vi "SC_schleife_init.vi"   [LabVIEW 2016]
uses:
  Oxford Software/Oxsoft/RAMP.LLB/RampTState.ctl
  Global/Global Variables/global.vi
  Global/Global Variables/Data_Display_global.vi
  Instrument_Setup.vi
types:
  T1 = typedef "RampTState.ctl" = enum16{"START", "RUN"}
  T2 = cluster{"ControlTITC":i8, "ControlTCh":i8, "SampleTITC":i8, "SampleTCh":i8}
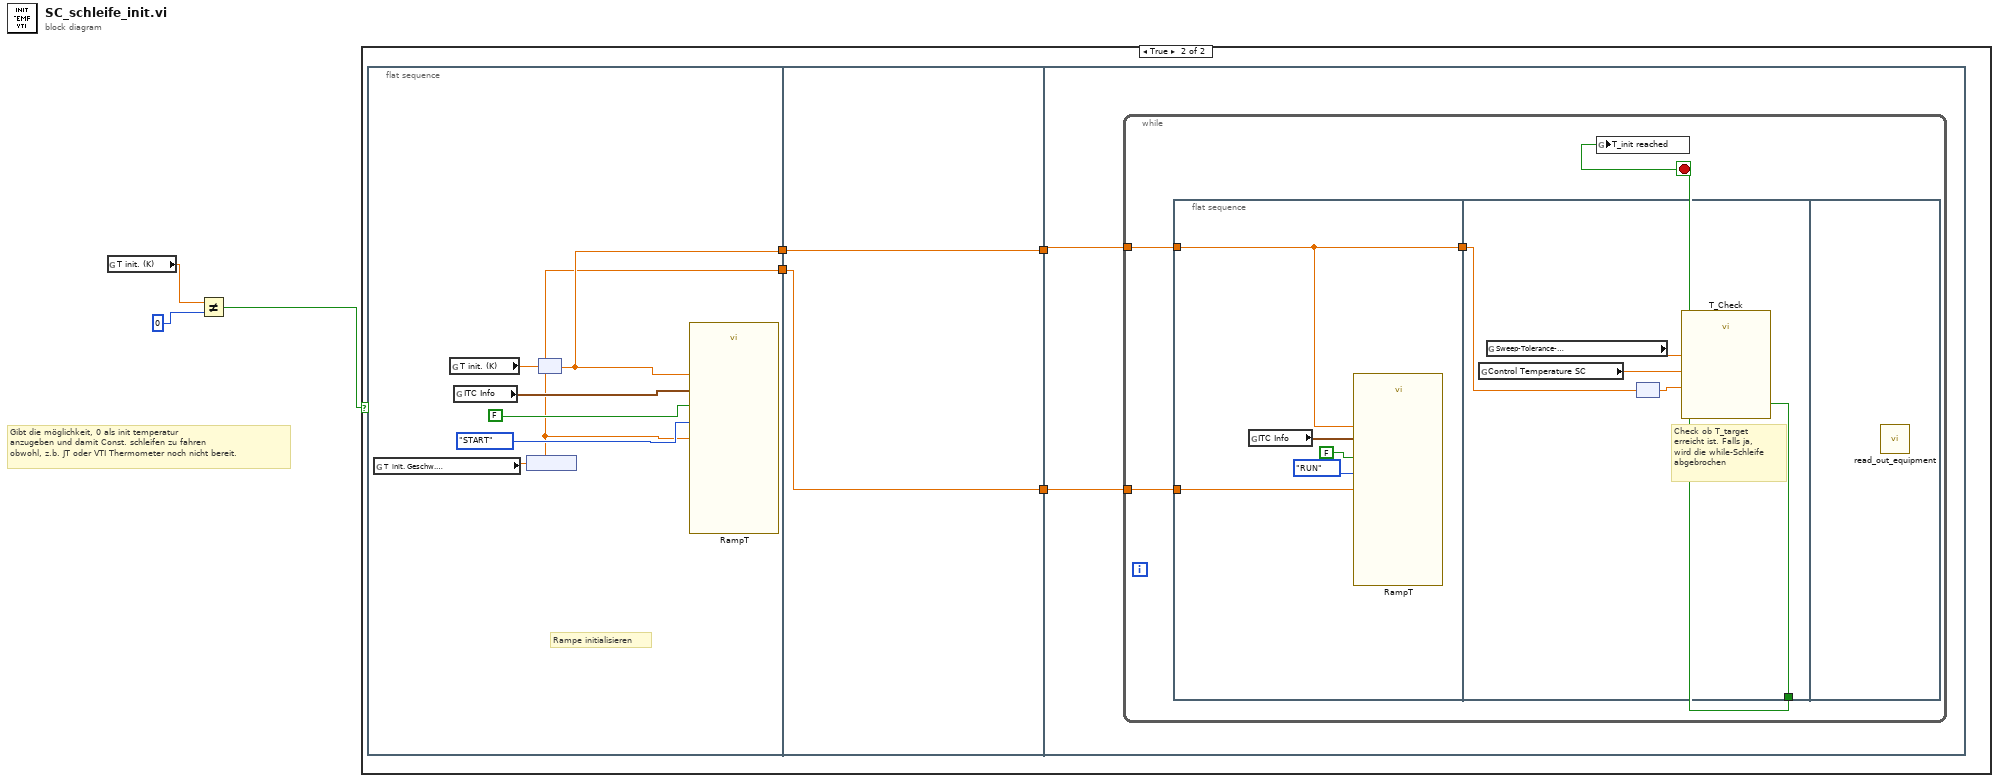
[diagram p0: block diagram]
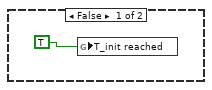
[diagram p2: hidden frame]
diagram:
  # "Gibt die möglichkeit, 0 als init temperatur \nanzugeben und damit Const. schleifen zu fahren\nobwohl, z.b. JT oder VTI Thermometer noch nicht bereit."
  n1 = global read "global.vi" "T init. (K)"() -> (w3:dbl)
  n2 = Not Equal?(x=w3, y=0) -> (x != y?=w1:bool)
  n3 = case shown="True" w1 {
    frame False {
      n4 = global write "Data_Display_global.vi" "T_init reached"(TRUE) -> ()
    }
    frame True {
      n5 = flat-sequence {
        tunnel: [w9] -> w8
        tunnel: [w10] -> w7
        tunnel: w8 -> [w16]
        tunnel: w7 -> [w17]
        tunnel: [w17] -> w6
        tunnel: [w16] -> w5
        tunnel: w6 -> [w19]
        tunnel: w5 -> [w18]
        frame #0 {
          # "Rampe initialisieren"
          n6 = global read "global.vi" "T  init. Geschw. \n(K/min)"() -> (w15:dbl)
          n7 = global read "global.vi" "T init. (K)"() -> (w14:dbl)
          n8 = global read "Instrument_Setup.vi" "ITC Info"() -> (w11:T2)
          n9 = node(w15) -> (w9:dbl[unit])
          n10 = node(w14) -> (w10:dbl[unit])
          n11 = call "RampT.vi"("ITC Info"=w11, "Rate"=w9, "Final Temperature"=w10, "JustReadTemperature"=FALSE, "RampTState"=RampTState."START") -> ()  [unwired: 5 out]
        }
        frame #1 {
        }
        frame #2 {
          n12 = while {
            tunnel: w19 -> [w23]
            tunnel: w18 -> [w20]
            stop <- w22 stop-if-true
            n13 = flat-sequence {
              tunnel: w23 -> [w25]
              tunnel: [w25] -> w21
              tunnel: w20 -> [w24]
              tunnel: [w31] -> w22
              tunnel: w21 -> [w33]
              frame #0 {
                n14 = global read "Instrument_Setup.vi" "ITC Info"() -> (w28:T2)
                n15 = call "RampT.vi"("ITC Info"=w28, "Rate"=w24, "Final Temperature"=w25, "JustReadTemperature"=FALSE, "RampTState"=RampTState."RUN") -> ()  [unwired: 5 out]
              }
              frame #1 {
                # "Check ob T_target\nerreicht ist. Falls ja,\nwird die while-Schleife\nabgebrochen"
                n16 = global read "Data_Display_global.vi" "Control Temperature SC"() -> (w29:dbl)
                n17 = global read "Instrument_Setup.vi" "Sweep-Tolerance-\nTemperature"() -> (w30:dbl)
                n18 = node(w33) -> (w32:dbl)
                n19 = call "T_Check.vi"("Sweep\nTolerance %"=w30, "T_target (K)"=w32, "T_in"=w29) -> ("= T target"=w31:bool)
              }
              frame #2 {
                n20 = call "read_out_equipment.vi"() -> ()  [unwired: 1 in]
              }
            }
            n21 = global write "Data_Display_global.vi" "T_init reached"(w22) -> ()
          }
        }
      }
    }
  }
